vi "fgv_tcp_remote.vi"(7 "cmd":T1=enum."init", 8 "error in":errorcluster, 9 "time-out":i32=3000, 10 "read byte":i32=3000, 11 "send data str":string) -> (0 "error out":errorcluster, 1 "remote_cmd":cluster{"cmp type":string, "content":string}, 2 "read bytes":i32, 3 "receive data str":string)   [LabVIEW 2019]
uses:
  Ctrl/tcp-srv.ctl
panel:
  out "content":string
  out "cmd":string
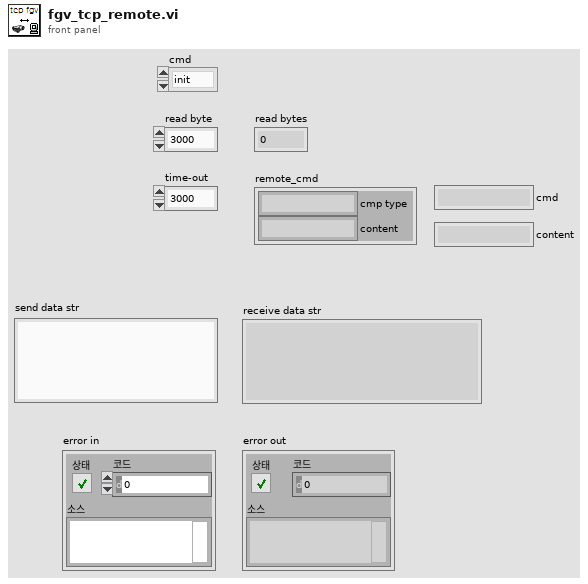
[diagram p1: front panel]
types:
  T1 = typedef "tcp-srv.ctl" = enum16{"read packet", "read header", "init", "read", "write", "close"}
  T2 = enum16{"Standard", "Buffered", "CRLF", "Immediate"}
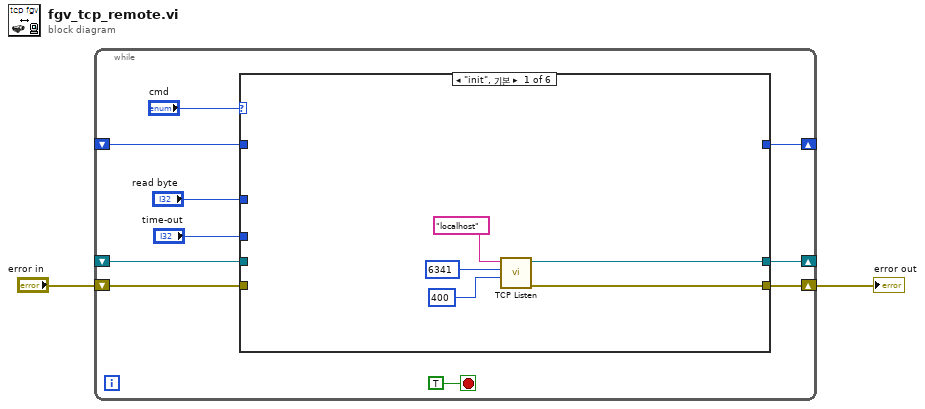
[diagram p0: block diagram]
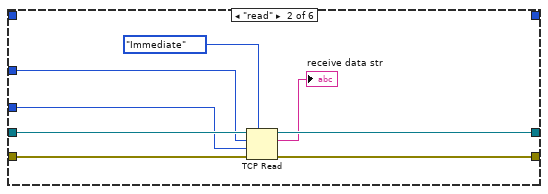
[diagram p2: hidden frame]
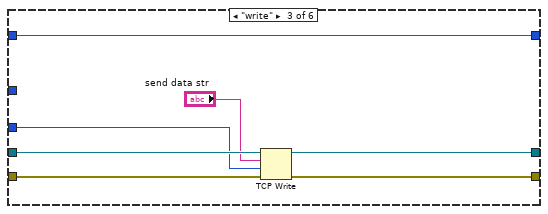
[diagram p3: hidden frame]
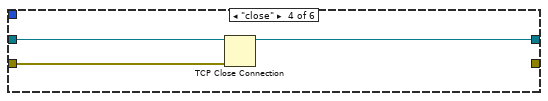
[diagram p4: hidden frame]
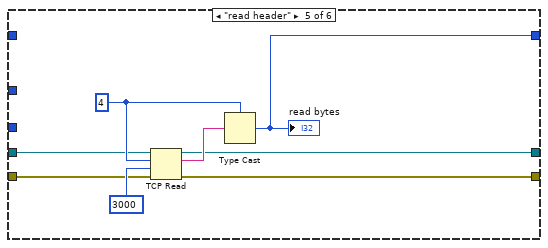
[diagram p5: hidden frame]
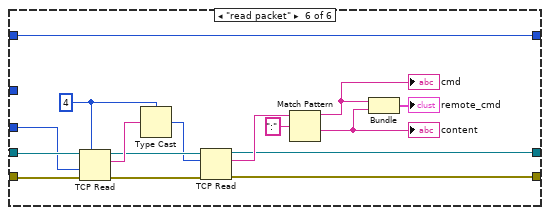
[diagram p6: hidden frame]
diagram:
  n1 = while {
    shift-right: [w10] -> _
    shift-left: _ -> [w9]
    shift-right: [w11] -> w1
    shift-left: "error in" -> [w8]
    shift-right: [w4] -> _
    shift-left: _ -> [w3]
    stop <- TRUE stop-if-true
    n2 = case shown="\"init\", 기본" "cmd" {
      tunnel: [w14 w24 w32 _ w38 w56] -> w11
      tunnel: [w13 w23 w31 w34 w37 w57] -> w10
      tunnel: w9 -> [_ w22 w30 w33 w40 w48]
      tunnel: w8 -> [_ w21 w29 w35 w39 w49]
      tunnel: "read byte" -> [_ w19 _ _ _ _]
      tunnel: "time-out" -> [_ w18 w27 _ _ w45]
      tunnel: [_ _ w26 _ w36 w52] -> w4
      tunnel: w3 -> [_ _ w26 _ _ w52]
      frame "init", Default {
        n3 = call <vilib>:"TCP Listen.vi"("timeout ms (wait forever: -1)"=400, "port"=u16 6341, "service name"="localhost") -> ("error out"=w14:errorcluster, "connection ID"=w13:refnum<k5>)  [unwired: 4 in, 3 out]
      }
      frame "read" {
        n4 = TCP Read(connection ID=w22, bytes to read=w19, error in (no error)=w21, 7:T2."Immediate" ("모드(standard)"), 9:w18) -> (connection ID out=w23:refnum<k5>, data out=→"receive data str":string, error out=w24:errorcluster)
      }
      frame "write" {
        n5 = TCP Write(connection ID=w30, data in="send data str", error in (no error)=w29, 9:w27) -> (connection ID out=w31:refnum<k5>, error out=w32:errorcluster)  [unwired: 1 out]
      }
      frame "close" {
        n6 = TCP Close Connection(connection ID=w33, error in (no error)=w35) -> (connection ID out=w34:refnum<k5>)  [unwired: 1 in, 1 out]
      }
      frame "read header" {
        w43 = 4 ("읽을 바이트")
        n7 = TCP Read(connection ID=w40, bytes to read=w43, error in (no error)=w39, 9:3000 ("타임아웃 ms (25000)")) -> (connection ID out=w37:refnum<k5>, data out=w42:string, error out=w38:errorcluster)  [unwired: 1 in]
        n8 = Type Cast(type=w43, x=w42) -> (*(type *) &x=w36:i32)
        "read bytes" <- w36
      }
      frame "read packet" {
        w50 = 4 ("읽을 바이트")
        n9 = TCP Read(connection ID=w48, bytes to read=w50, error in (no error)=w49, 9:w45) -> (connection ID out=w46:refnum<k5>, data out=w51:string, error out=w47:errorcluster)  [unwired: 1 in]
        n10 = Type Cast(type=w50, x=w51) -> (*(type *) &x=w44:i32)
        n11 = TCP Read(connection ID=w46, bytes to read=w44, error in (no error)=w47) -> (connection ID out=w57:refnum<k5>, data out=w58:string, error out=w56:errorcluster)  [unwired: 2 in]
        n12 = Match Pattern(string=w58, regular expression=":" ("정규식")) -> (before substring=w55:string, after substring=w54:string)  [unwired: 1 in, 2 out]
        "cmd" <- w55
        "content" <- w54
        n13 = Bundle("data out"=w55, "data out"=w54) -> (→"remote_cmd":cluster{"data out":string, "data out":string})  [unwired: 1 in]
      }
    }
  }
  "error out" <- w1
